vi "Potting Data - TBM TBM.vi"(8 "error in":errorcluster, 10 "TBM-TBM Selection":T6, 11 "TBM-TBM Data":T2) -> (0 "error out":errorcluster, 3 "Potting Lines":T1[](array[typedef]))   [LabVIEW 2011]
uses:
  Shared Components/Utils/Type Definitions/Multi-Fiducial Image.ctl
  Shared Components/Vec3d Class/Vec3d Class.lvclass
  Shared Components/Utils/Type Definitions/Physical Image.ctl
  <vilib>/vision/Image Controls.llb/IMAQ Image.ctl
  Shared Components/Utils/Type Definitions/Fiducial with Source.ctl
  Shared Components/Utils/Type Definitions/3d Line.ctl
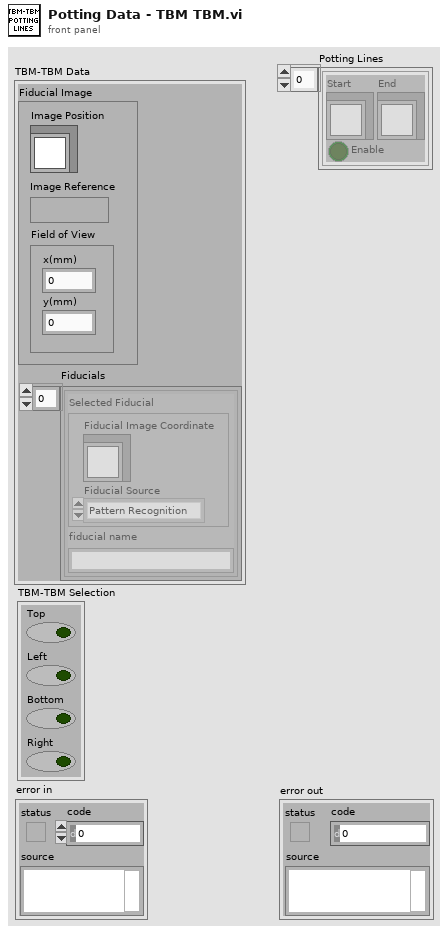
[diagram p1: front panel]
types:
  T1 = typedef "3d Line.ctl" = cluster{"Start":refnum<class "Vec3d Class.lvclass">, "End":refnum<class "Vec3d Class.lvclass">, "Enable":bool}
  T2 = typedef "Multi-Fiducial Image.ctl" = cluster{"Fiducial Image":T3, "Fiducials":cluster{"Selected Fiducial":T5, "fiducial name":string}[]}
  T3 = typedef "Physical Image.ctl" = cluster{"Image Position":refnum<class "Vec3d Class.lvclass">, "Image Reference":T4, "Field of View":cluster{"x(mm)":dbl, "y(mm)":dbl}}
  T4 = typedef "IMAQ Image.ctl" = refnum<image>
  T5 = typedef "Fiducial with Source.ctl" = cluster{"Fiducial Image Coordinate":refnum<class "Vec3d Class.lvclass">, "Fiducial Source":enum16{"Pattern Recognition", "User", "Error", "Default"}}
  T6 = cluster{"Top":bool, "Left":bool, "Bottom":bool, "Right":bool}
  T7 = cluster{"Selected Fiducial":T5, "fiducial name":string}[]
  T8 = cluster{"Selected Fiducial":T5, "fiducial name":string}
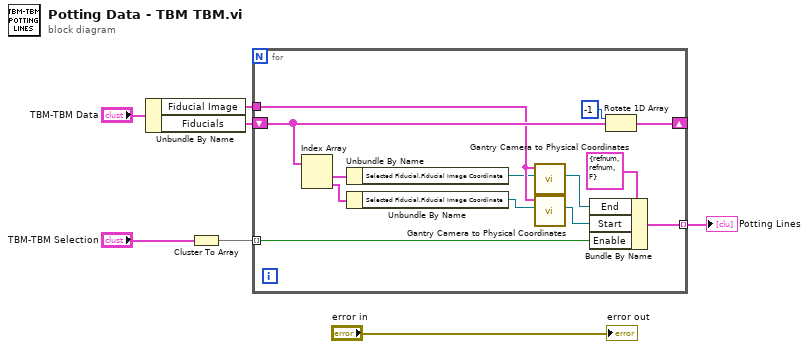
[diagram p0: block diagram]
diagram:
  n1 = Unbundle By Name("TBM-TBM Data") -> ("Fiducial Image"=w3:T3, "Fiducials"=w4:T7)
  n2 = Cluster To Array(cluster="TBM-TBM Selection") -> (array=w5:bool[])
  n3 = for {
    tunnel: w5 -> [w8] mode=indexing
    shift-right: [w18] -> _
    shift-left: w4 -> [w19]
    tunnel: w3 -> [w17]
    tunnel: [w9] -> w2 mode=indexing
    n4 = Index Array(array=w19) -> (element #1=w15:T8, element #2=w16:T8)  [unwired: 2 in]
    n5 = Unbundle By Name(w15) -> ("Selected Fiducial.Fiducial Image Coordinate"=w13:refnum<class "Vec3d Class.lvclass">)
    n6 = Unbundle By Name(w16) -> ("Selected Fiducial.Fiducial Image Coordinate"=w12:refnum<class "Vec3d Class.lvclass">)
    n7 = call "Gantry Camera to Physical Coordinates.vi"("Image Coordinate"=w13, "Physical Image"=w17) -> ("Global Coordinate"=w11:refnum<class "Vec3d Class.lvclass">)  [unwired: 7 in, 2 out]
    n8 = call "Gantry Camera to Physical Coordinates.vi"("Image Coordinate"=w12, "Physical Image"=w17) -> ("Global Coordinate"=w10:refnum<class "Vec3d Class.lvclass">)  [unwired: 7 in, 2 out]
    n9 = Bundle By Name(cluster=T1 {"Start"=refnum, "End"=refnum, "Enable"=FALSE} ("3D Line"), "End"=w11, "Start"=w10, "Enable"=w8) -> (w9:T1)
    n10 = Rotate 1D Array(1:w19, 2:-1 ("n")) -> (0:w18:T7)
  }
  "Potting Lines" <- w2
  "error out" <- "error in"
